vi "Add_Props_Text.vi"(10 "Text Properties":T2={"Color"=0, "Background Color"=2147483647, "Font Size (points)"=0, "Font Style"=enum."Automatic", "Rotation Angle"=nan} {"Background Color" items=["Automatic"=2147483647, "Black"=0, "White"=16777215, "Red"=16711680, "Green"=2263842, "Blue"=255, "Cyan"=65535, "Magenta"=16711935, "Yellow"=16776960]; "Font Size (points)" items=["Automatic"=0, "XX-Small"=-1, "X-Small"=-2, "Small"=-3, "Medium"=-4, "Large"=-5, "X-Large"=-6, "XX-Large"=-7]; "Color" items=["Automatic"=2147483647, "Black"=0, "White"=16777215, "Red"=16711680, "Green"=2263842, "Blue"=255, "Cyan"=65535, "Magenta"=16711935, "Yellow"=16776960]}, 11 "Keyword Array":T1[](array[typedef])) -> (3 "Keyword Array Out":T1[](array[typedef]))   [LabVIEW 2013, in "Advanced Plotting Toolkit.lvlib"]
uses:
  Advanced Plotting Toolkit.lvlib
  properties/Text.ctl
  typedefs/PlotColor.ctl
  properties/Text_FontSize.ctl
  properties/Text_FontStyle.ctl
  KeyValue.ctl
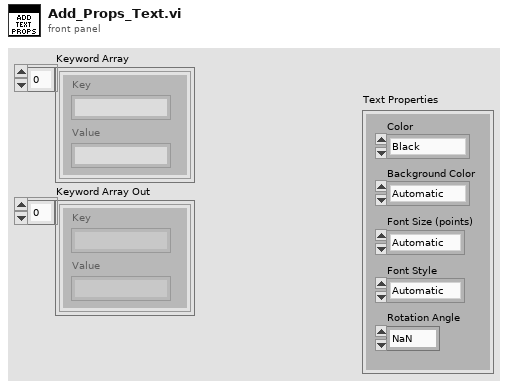
[diagram p1: front panel]
types:
  T1 = typedef "Advanced Plotting Toolkit.lvlib/KeyValue.ctl" = cluster{"Key":string, "Value":string}
  T2 = typedef "Advanced Plotting Toolkit.lvlib/Text.ctl" = cluster{"Color":T3, "Background Color":T3, "Font Size (points)":T4, "Font Style":T5, "Rotation Angle":dbl}
  T3 = typedef "Advanced Plotting Toolkit.lvlib/PlotColor.ctl" = u32
  T4 = typedef "Advanced Plotting Toolkit.lvlib/Text_FontSize.ctl" = i32
  T5 = typedef "Advanced Plotting Toolkit.lvlib/Text_FontStyle.ctl" = enum16{"Automatic", "Normal", "Italic", "Bold"}
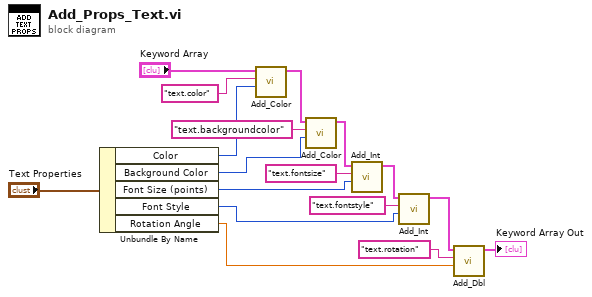
[diagram p0: block diagram]
diagram:
  n1 = Unbundle By Name("Text Properties") -> ("Color"=w14:T3, "Background Color"=w11:T3, "Font Size (points)"=w10:T4, "Font Style"=w2:T5, "Rotation Angle"=w5:dbl)
  n2 = call "Add_Color.vi"("Color"=w14, "Key"="text.color", "Keyword Array"="Keyword Array") -> ("Keyword Array Out"=w12:T1[])  [unwired: 8 in]
  n3 = call "Add_Color.vi"("Color"=w11, "Key"="text.backgroundcolor", "Keyword Array"=w12) -> ("Keyword Array Out"=w9:T1[])  [unwired: 8 in]
  n4 = call "Add_Int.vi"("Value"=w10, "Key"="text.fontsize", "Keyword Array"=w9) -> ("Keyword Array Out"=w7:T1[])  [unwired: 8 in]
  n5 = call "Add_Int.vi"("Value"=w2, "Key"="text.fontstyle", "Keyword Array"=w7) -> ("Keyword Array Out"=w4:T1[])  [unwired: 8 in]
  n6 = call "Add_Dbl.vi"("Value"=w5, "Key"="text.rotation", "Keyword Array"=w4) -> ("Keyword Array Out"=→"Keyword Array Out":T1[])  [unwired: 8 in]
